vi "LoadData.vi"(5 "Path":refnum<vi>) -> (0 "gap photons":u32, 1 "invalid photons":u32, 2 "total":u32)   [LabVIEW 2009]
panel:
  out "% done":dbl(slide) scale=0.0..100.0
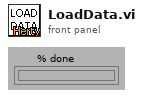
[diagram p1: front panel]
types:
  T1 = typedef "FIFOSettings_BH.ctt" = cluster{"Measurement":cluster{"Binning (ms)":sgl, "External Trigger Condition":u16, "Stop Condition:":u16, "Stop Count":dbl, "Buffer Size (Photons)":u16, "No of Channels":u16, "Ext Latch Delay":i16}, "ADC":cluster{"Module":u16, "ADC Resolution":i32, "Dither Range":i16, "Count Increment":i16, "Macro Time Clock":i16}, "SYNC":cluster{"SYNC ZC Level (mV)":sgl, "SYNC Freq Divider":i16, "SYNC Holdoff (ns)":sgl, "SYNC Threshold (mV)":sgl}, "TAC":cluster{"TAC Range (ns)":sgl, "TAC Gain":i16, "TAC Offset (%)":sgl, "TAC Limit Low (%)":sgl, "TAC Limit High (%)":sgl}, "CFD":cluster{"CFD Limit Low (mV)":sgl, "CFD Limit High (mV)":sgl, "CFD ZC Level (mV)":sgl, "CFD Holdoff (ns)":sgl}}
  T2 = cluster{"router channels":u8[], "macro times":dbl[], "micro times":u16[], "invalid times":dbl[], "gap times":dbl[]}
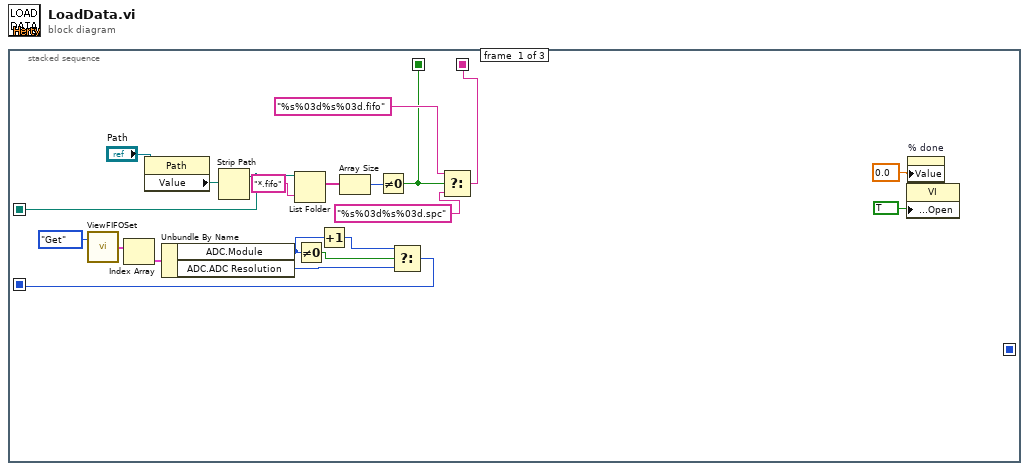
[diagram p0: block diagram]
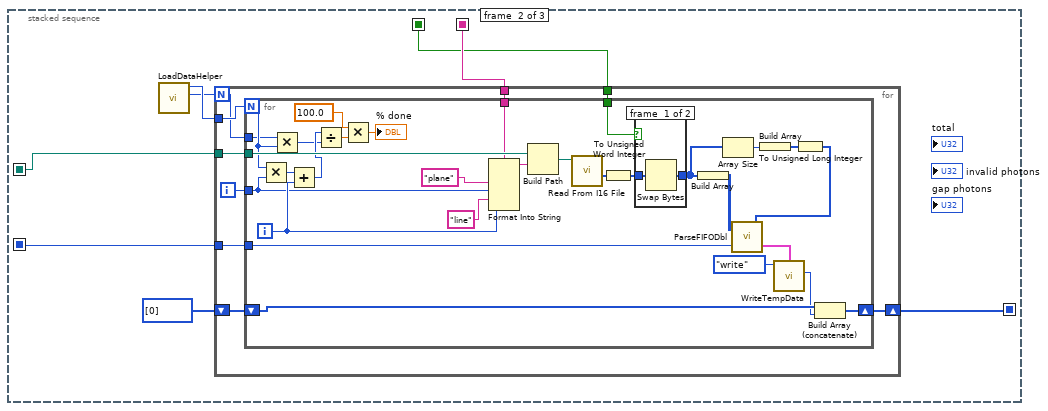
[diagram p2: hidden frame]
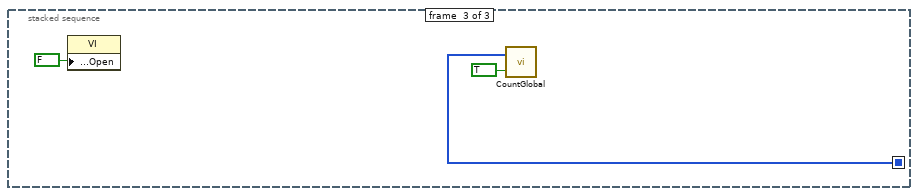
[diagram p4: hidden frame]
diagram:
  n1 = stacked-sequence {
    seq-local: [_ w27 _] -> [_ _ w73]
    seq-local: [w12 _ _] -> [_ w24 _]
    seq-local: [w2 _ _] -> [_ w23 _]
    seq-local: [w8 _ _] -> [_ w22 _]
    seq-local: [w1 _ _] -> [_ w21 _]
    frame #0 {
      n2 = call "ViewFIFOSet.vi"("Enum"=enum16{"Display", "change", "Get", "Set"}."Get") -> ("FIFO Settings (Array)"=w17:T1[])  [unwired: 1 in]
      n3 = Index Array(array=w17) -> (element=w16:T1)  [unwired: 1 in]
      n4 = property on="Property Node" class="Path"(reference="Path") -> ("Value"=w10:path)  [unwired: 1 in, 2 out]
      n5 = Unbundle By Name(w16) -> ("ADC.Module"=w13:u16, "ADC.ADC Resolution"=w15:i32)
      n6 = Strip Path(path=w10) -> (stripped path=w8:path)  [unwired: 1 out]
      n7 = List Folder(path=w8, pattern="*.fifo") -> (filenames=w6:string[])  [unwired: 2 in, 3 out]
      n8 = Not Equal To 0?(x=w13) -> (x != 0?=w14:bool)
      n9 = Increment(x=w13) -> (x+1=w11:u16)
      n10 = Array Size(array=w6) -> (size(s)=w5:i32)
      n11 = Not Equal To 0?(x=w5) -> (x != 0?=w1:bool)
      n12 = Select(t=w11, s=w14, f=w15) -> (s? t:f=w12:i32)
      n13 = Select(t="%s%03d%s%03d.fifo" ("format string"), s=w1, f="%s%03d%s%03d.spc" ("format string")) -> (s? t:f=w2:string)
      n14 = property class="VI"("Front Panel Window:Open"=TRUE) -> ()  [unwired: 2 in, 2 out]
      n15 = property on="% done" class="Slide (strict)"("Value"=0.0 ("% done")) -> ()  [unwired: 2 in, 2 out]
    }
    frame #1 {
      n16 = call "LoadDataHelper.vi"() -> ("planes"=w25:u32, "lines"=w26:u32)  [unwired: 7 in, 3 out]
      n17 = for {
        N: w25 -> [w31]
        tunnel: w26 -> [w34]
        tunnel: w22 -> [w37]
        tunnel: w24 -> [w35]
        shift-right: [w32] -> w27
        shift-left: i32[] [0] -> [w33]
        tunnel: w23 -> [w30]
        tunnel: w21 -> [w29]
        i -> [w36]
        n18 = for {
          N: w34 -> [w52]
          tunnel: w37 -> [w67]
          tunnel: w36 -> [w55]
          tunnel: w35 -> [w49]
          shift-right: [w65] -> w32
          shift-left: w33 -> [w66]
          tunnel: w31 -> [w51]
          tunnel: w30 -> [w42]
          tunnel: w29 -> [w41]
          i -> [w56]
          n19 = Multiply(x=w52, y=w55) -> (x*y=w53:i32)
          n20 = Multiply(x=w51, y=w52) -> (x*y=w50:i32)
          n21 = Add(x=w53, y=w56) -> (x+y=w54:i32)
          n22 = Divide(x=w54, y=w50) -> (x/y=w64:dbl)
          n23 = Multiply(x=100.0, y=w64) -> (x*y=→"% done":dbl)
          n24 = Format Into String(format string=w42, "plane", w55, "line", w56) -> (resulting string=w59:string)  [unwired: 2 in, 1 out]
          n25 = Build Path(base path=w67, name or relative path=w59) -> (appended path=w58:path)
          n26 = call "Read From I16 File.vi"("file path (dialog if empty)"=w58) -> ("1D array"=w57:i16[])  [unwired: 6 in, 4 out]
          n27 = To Unsigned Word Integer(number=w57) -> (unsigned 16bit integer=w44:u16[])
          n28 = case shown="False" w41 {
            tunnel: w44 -> [w69 w70]
            tunnel: [w68 w70] -> w43
            frame #0 {
              n29 = Swap Bytes(anything=w69) -> (byte swapped=w68:u16[])
            }
            frame #1 {
            }
          }
          n30 = Build Array(w43) -> (w48:u16[][])
          n31 = Array Size(array=w43) -> (size(s)=w47:i32)
          n32 = Build Array(w47) -> (w46:i32[])
          n33 = To Unsigned Long Integer(number=w46) -> (unsigned 32bit integer=w45:u32[])
          n34 = call "ParseFIFODbl.vi"("photoncount"=w45, "SPC Format"=w49, "FIFO rawdata"=w48) -> ("rawdata"=w39:T2)
          n35 = call "WriteTempData.vi"("rawdata"=w39, "Enum"=enum16{"create new", "write", "close"}."write") -> ("offset"=w38:i32)  [unwired: 3 in, 1 out]
          n36 = Build Array (concatenate)(w66, w38) -> (w65:i32[])
        }
      }
    }
    frame #2 {
      n37 = property class="VI"("Front Panel Window:Open"=FALSE) -> ()  [unwired: 2 in, 2 out]
      n38 = call "CountGlobal.vi"("changed?"=TRUE, "count"=w73) -> ()  [unwired: 1 in, 1 out]
    }
  }
